vi "RoundAndRescale_subvi.vi"(6 "maxX":dbl, 9 "minX":dbl, 10 "all rows":dbl[](array[numeric]), 11 "numbins":dbl) -> (3 "RoundedArray":dbl[](array[numeric]))   [LabVIEW 2019]
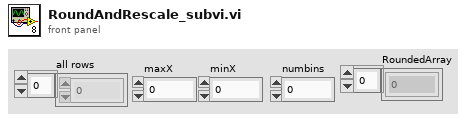
[diagram p1: front panel]
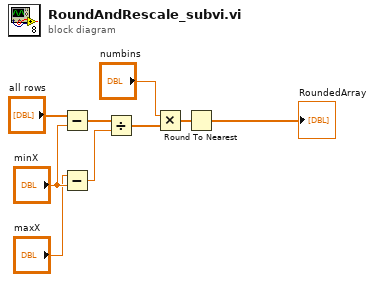
[diagram p0: block diagram]
diagram:
  n1 = Subtract(x="all rows", y="minX") -> (x-y=w5:dbl[])
  n2 = Subtract(x="maxX", y="minX") -> (x-y=w4:dbl)
  n3 = Divide(x=w5, y=w4) -> (x/y=w6:dbl[])
  n4 = Multiply(x="numbins", y=w6) -> (x*y=w7:dbl[])
  n5 = Round To Nearest(number=w7) -> (nearest integer value=→"RoundedArray":dbl[])
